vi "Write Time Stamp.vi"(8 "error in (no error)":errorcluster, 10 "Time Stamp":timestamp, 11 "RDS State in":refnum<class "RDS State.lvclass">) -> (0 "error out":errorcluster, 3 "RDS State out":refnum<class "RDS State.lvclass">)   [LabVIEW 2015, in "RDS Child Messages.lvlib" / "RDS State.lvclass"]
uses:
  RDS State.lvclass
  RDS State.lvclass/RDS State.ctl
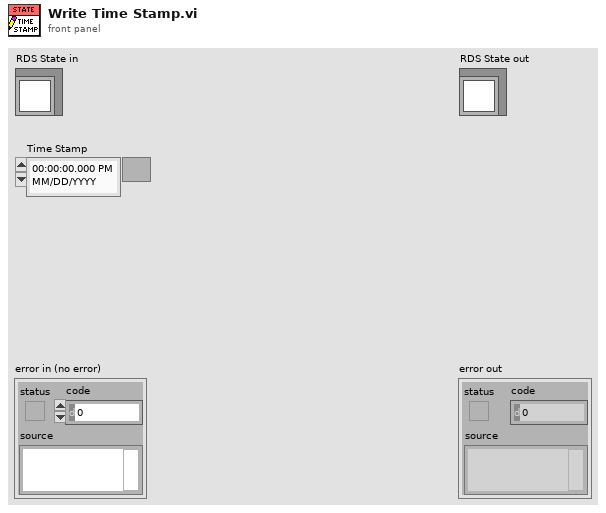
[diagram p1: front panel]
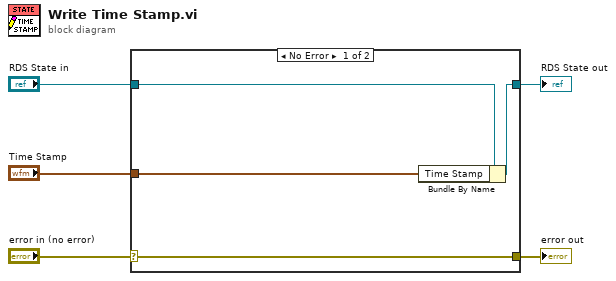
[diagram p0: block diagram]
diagram:
  n1 = case shown="No Error" "error in (no error)" {
    selector: "error in (no error)" -> [w9 w10]
    tunnel: [w9 w10] -> w4
    tunnel: [w7 w11] -> w2
    tunnel: "RDS State in" -> [w8 w11]
    tunnel: "Time Stamp" -> [w6 _]
    frame No Error {
      n2 = Bundle By Name(cluster=w8, "Time Stamp"=w6) -> (w7:refnum<class "RDS State.lvclass">)
    }
    frame Error {
    }
  }
  "error out" <- w4
  "RDS State out" <- w2
